vi "S2C_FORNAX_Proc_Launch.vi"(8 "Error In":errorcluster, 10 "Timeout":dbl, 11 "Data":string) -> (0 "Error Out":errorcluster, 3 "Result":string)   [LabVIEW 2015]
uses:
  S2C_FORNAX_Proc_Globals.vi
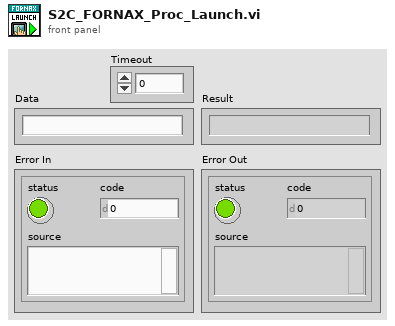
[diagram p1: front panel]
types:
  T1 = cluster{"Path":string, "Port":i32, "Version":i32}
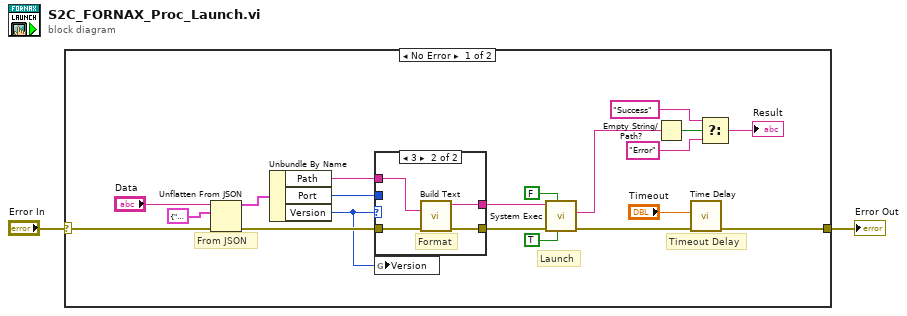
[diagram p0: block diagram]
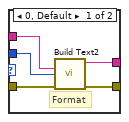
[diagram p2: hidden frame]
diagram:
  n1 = case shown="No Error" "Error In" {
    selector: "Error In" -> [w11 w32]
    tunnel: [w10 w32] -> w1
    frame No Error {
      # "Timeout Delay"
      # "From JSON"
      # "Launch"
      n2 = Unflatten From JSON(JSON string="Data", type and defaults=T1 {"Path"="", "Port"=0, "Version"=0}, error in (no error)=w11) -> (value=w13:T1, error out=w14:errorcluster)  [unwired: 4 in]
      n3 = Unbundle By Name(w13) -> ("Path"=w5:string, "Port"=w4:i32, "Version"=w3:i32)
      n4 = case shown="3" w3 {
        tunnel: [w27 w31] -> w22
        tunnel: [w26 w30] -> w21
        tunnel: w14 -> [w25 w29]
        tunnel: w5 -> [w24 w28]
        tunnel: w4 -> [w23 _]
        frame 0, Default {
          # "Format"
          n5 = call "Build Text2"("Path"=w24, "Port"=w23, "error in (no error)"=w25) -> ("Result"=w27:string, "error out"=w26:errorcluster)  [unwired: 11 in]
        }
        frame 3 {
          # "Format"
          n6 = call "Build Text"("FornaxPath"=w28, "error in (no error)"=w29) -> ("Result"=w31:string, "error out"=w30:errorcluster)  [unwired: 12 in]
        }
      }
      n7 = global write "S2C_FORNAX_Proc_Globals.vi" "Version"(w3) -> ()
      n8 = call <vilib>:"System Exec.vi"("run minimized? (F)"=TRUE, "wait until completion? (T)"=FALSE, "error in (no error)"=w21, "command line"=w22) -> ("error out"=w12:errorcluster, "standard error"=w15:string)  [unwired: 4 in, 2 out]
      n9 = Empty String/Path?(string/path=w15) -> (empty?=w16:bool)
      n10 = call "Time Delay"("error in (no error)"=w12, "Delay Time (s)"="Timeout") -> ("error out"=w10:errorcluster)  [unwired: 9 in]
      n11 = Select(t="Success", s=w16, f="Error") -> (s? t:f=→"Result":string)
    }
    frame Error {
    }
  }
  "Error Out" <- w1
